vi "Post_AuthenticationCode_Request.vi"(8 "error in (no error)":errorcluster, 11 "OneNote in":refnum<class "OneNote.lvclass">) -> (0 "error out":errorcluster, 3 "OneNote out":refnum<class "OneNote.lvclass">)   [LabVIEW 2016, in "OneNote.lvclass"]
uses:
  OneNote.lvclass
  OneNote.lvclass/OneNote.ctl
  <vilib>/httpClient/POSTBuffer.vi
  <vilib>/httpClient/LabVIEWHTTPClient.lvlib
  <vilib>/addons/_JKI.lib/Serialization/JSON/JKI JSON Serialization.lvlib
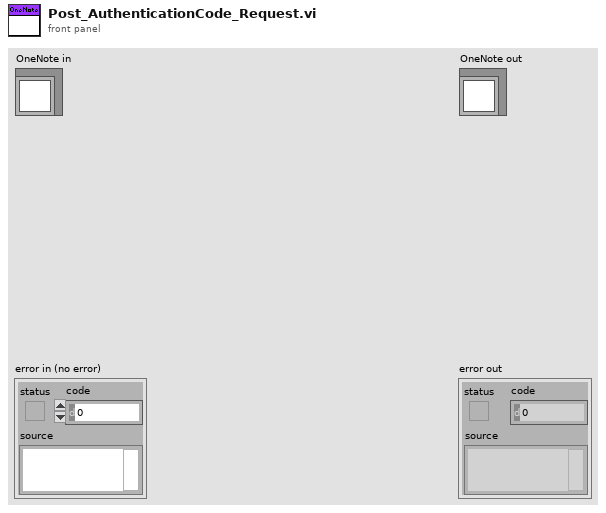
[diagram p1: front panel]
types:
  T1 = cluster{"token_type":string, "scope":string, "access_token":string, "refresh_token":string, "user_id":string, "expires_in":i32}
  T2 = typedef "LabVIEWHTTPClient.lvlib/ClientHandle.ctl" = refnum<k1>
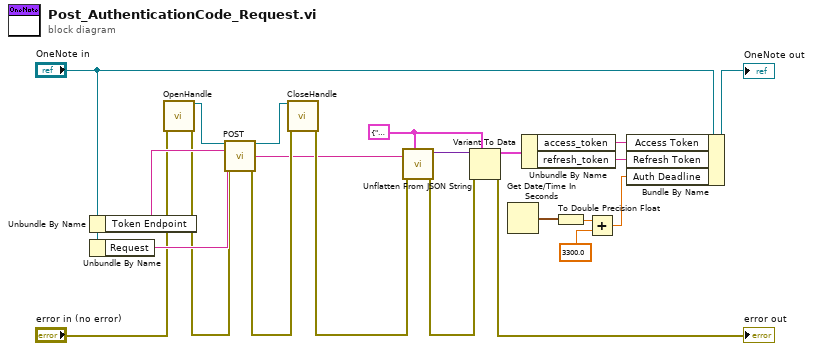
[diagram p0: block diagram]
diagram:
  w16 = T1 {"token_type"="", "scope"="", "access_token"="", "refresh_token"="", "user_id"="", "expires_in"=0}
  n1 = Unbundle By Name("OneNote in") -> ("Token Endpoint"=w20:string)
  n2 = Unbundle By Name("OneNote in") -> ("Request"=w19:string)
  n3 = call <vilib>:"OpenHandle.vi"("error in (no error)"="error in (no error)") -> ("client handle out"=w22:T2, "error out"=w18:errorcluster)  [unwired: 13 in]
  n4 = call-poly <vilib>:"POST.vi"("client handle"=w22, "url"=w20, "buffer"=w19, "error in (no error)"=w18) -> ("client handle out"=w21:T2, "body"=w5:string, "error out"=w17:errorcluster)  [unwired: 8 in, 1 out]
  n5 = call <vilib>:"CloseHandle.vi"("client handle"=w21, "error in (no error)"=w17) -> ("error out"=w11:errorcluster)  [unwired: 13 in]
  n6 = call <vilib>:"Unflatten From JSON String.vi"("Type and Defaults"=w16, "error in (no error)"=w11, "JSON String"=w5) -> ("error out"=w10:errorcluster, "Variant"=w15:variant)  [unwired: 7 in]
  n7 = Variant To Data(error in=w10, type=w16, Variant=w15) -> (data=w14:T1, error out=→"error out":errorcluster)
  n8 = Get Date/Time In Seconds() -> (seconds since 1Jan1904=w7:timestamp)
  n9 = Unbundle By Name(w14) -> ("access_token"=w13:string, "refresh_token"=w12:string)
  n10 = To Double Precision Float(number=w7) -> (double precision float=w8:dbl)
  n11 = Add(x=w8, y=3300.0) -> (x+y=w6:dbl)
  n12 = Bundle By Name(cluster="OneNote in", "Access Token"=w13, "Refresh Token"=w12, "Auth Deadline"=w6) -> (→"OneNote out":refnum<class "OneNote.lvclass">)
